vi "SuppressDAQError.vi"(6 "error IO":errorcluster) -> (0 "Error Out":errorcluster, 1 "Error Filtered?":bool)   [LabVIEW 2013, in "main.lvlib"]
uses:
  main.lvlib
  <userlib>/_OpenG.lib/error/error.llb/Filter Error Codes (Array)__ogtk.vi
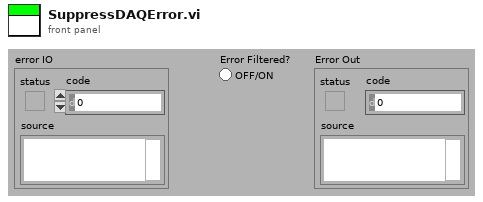
[diagram p1: front panel]
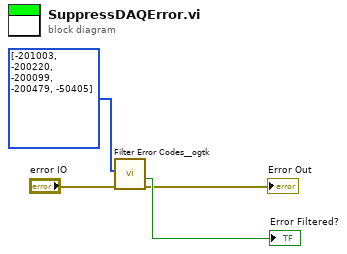
[diagram p0: block diagram]
diagram:
  n1 = call-poly <userlib>:"Filter Error Codes__ogtk.vi"("Error In"="error IO", "Error Codes to Filter"=i32[] [-201003, -200220, -200099, -200479, -50405]) -> ("Error Out"=→"Error Out":errorcluster, "Error Filtered?"=→"Error Filtered?":bool)  [unwired: 7 in, 1 out]
